vi "long_test_2.vi"(9 "string":string="tmp\\all_2.lvm", 10 "Instrument VISA in":T1={"AWG VISA"="81160A", "Oscilloscope  VISA "="DSO80204B", "Integration Board IP"="172.16.7.43", "connection ID"=refnum, "report out"=refnum, "report file path"=path "D:/CTA/Data_test"}, 11 "error in (no error)":errorcluster) -> (3 "error out":errorcluster)   [LabVIEW 2009]
uses:
  <vilib>/Utility/NIReport.llb/NI_report.lvclass
  <vilib>/Analysis/NI_AALBase.lvlib
panel:
  out "Numeric":i32
  out "atenuation":dbl[](array[numeric])
  out "clipping":dbl[](array[numeric])
  out "channel":dbl[](array[numeric])
  out "XY Graph":cluster{dbl[], dbl[]}[](graph)
  out "XY Graph 2":cluster{dbl[], dbl[]}[](graph)
  out "mean value 2":dbl=711.9915188935893
  in  "stop":bool
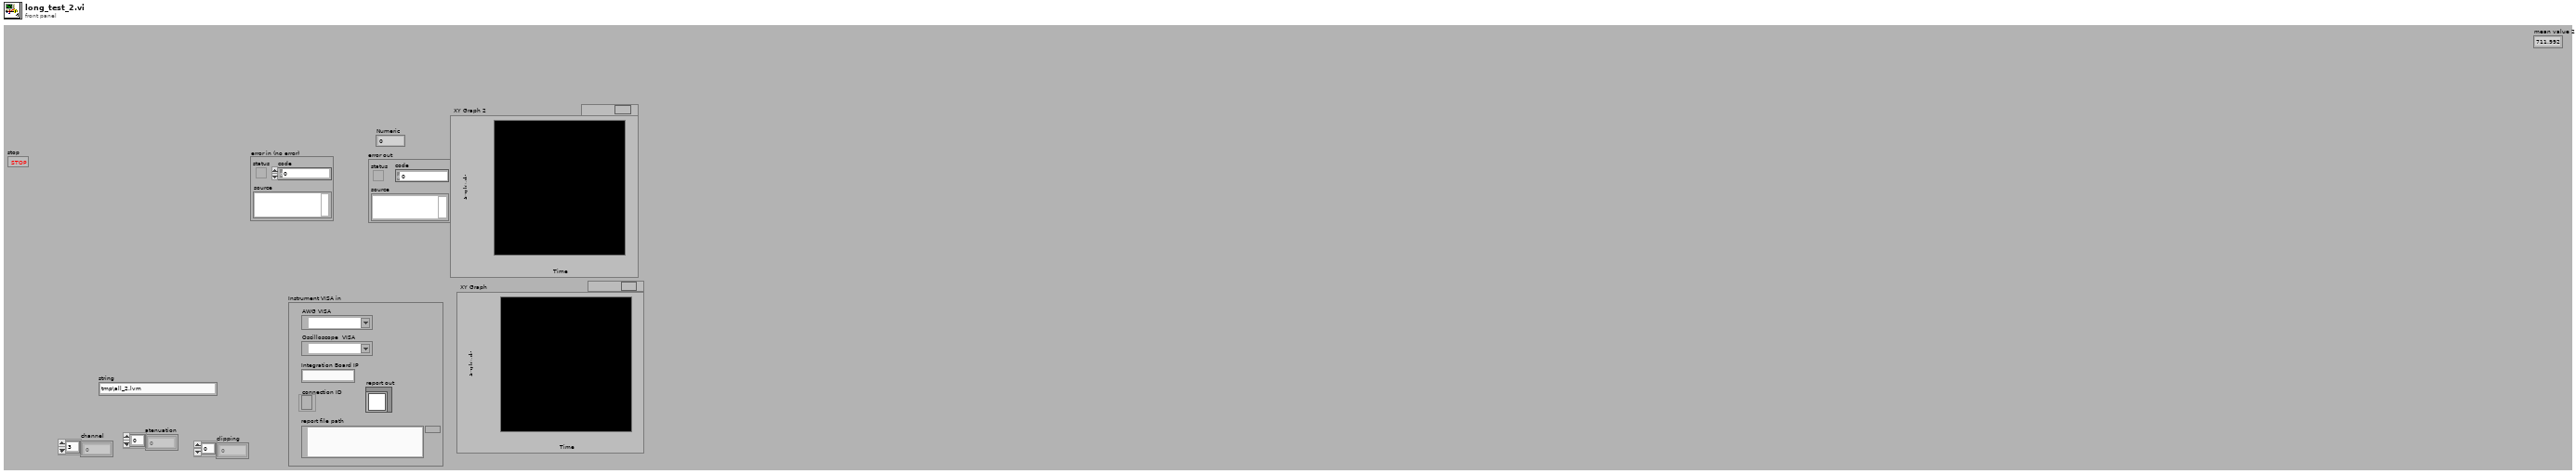
[diagram p1: front panel]
types:
  T1 = cluster{"AWG VISA":refnum<visa-resource-name>, "Oscilloscope  VISA ":refnum<visa-resource-name>, "Integration Board IP":string, "connection ID":refnum<k5>, "report out":refnum<class "NI_report.lvclass">, "report file path":path}
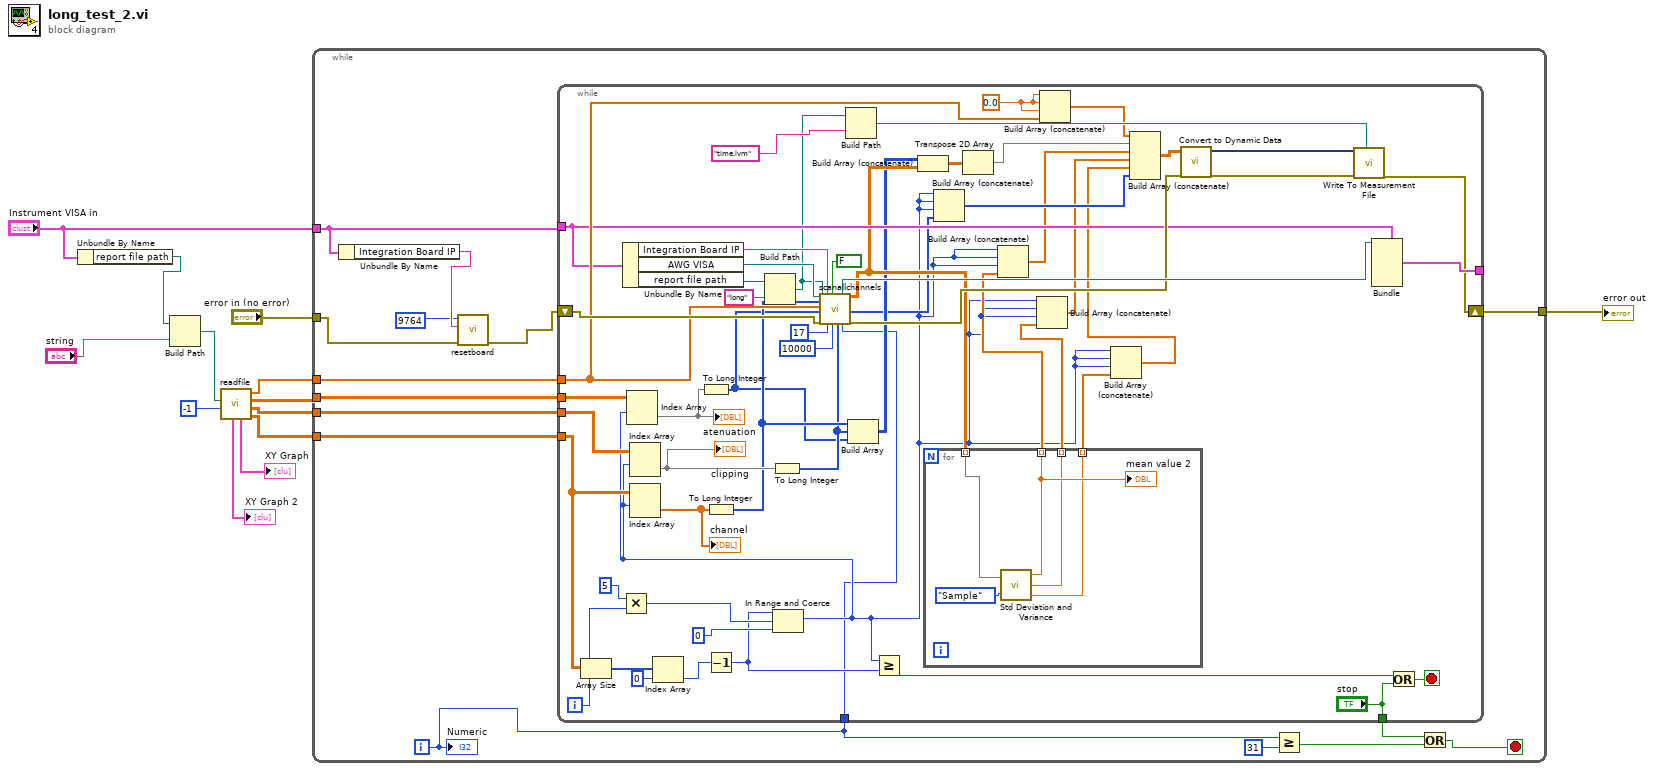
[diagram p0: block diagram]
diagram:
  n1 = Unbundle By Name("Instrument VISA in") -> ("report file path"=w5:path)
  n2 = Build Path(base path=w5, name or relative path="string") -> (appended path=w4:path)
  n3 = call "readfile.vi"("count"=-1, "file (use dialog)"=w4) -> ("channels"=w8:dbl[][], "clipping"=w7:dbl[][], "attenuator"=w6:dbl[][], "voltage"=w10:dbl[], "XY Graph"=→"XY Graph":cluster{dbl[], dbl[]}[], "XY Graph 2"=→"XY Graph 2":cluster{dbl[], dbl[]}[])  [unwired: 4 in]
  n4 = while {
    tunnel: w10 -> [w28]
    tunnel: "Instrument VISA in" -> [w21]
    tunnel: w8 -> [w27]
    tunnel: w7 -> [w26]
    tunnel: w6 -> [w25]
    tunnel: [w20] -> w2
    tunnel: "error in (no error)" -> [w19]
    i -> [w18]
    stop <- w14 stop-if-true
    n5 = Unbundle By Name(w21) -> ("Integration Board IP"=w24:string)
    n6 = call "resetboard.vi"("error in (no error)"=w19, "address"=w24, "remote port or service name"=u16 9764) -> ("error out"=w23:errorcluster)  [unwired: 7 in, 1 out]
    n7 = while {
      tunnel: w28 -> [w71]
      tunnel: w21 -> [w68]
      tunnel: [w69] -> _
      shift-right: [w65] -> w20
      shift-left: w23 -> [w75]
      tunnel: w27 -> [w62]
      tunnel: w26 -> [w63]
      tunnel: w25 -> [w64]
      tunnel: ["stop"] -> w16
      tunnel: w18 -> [w29]
      i -> [w36]
      stop <- w59 stop-if-true
      w76 = 0.0 ("element")
      n8 = Array Size(array=w62) -> (size(s)=w61:i32[])
      n9 = Multiply(x=5 ("index"), y=w36) -> (x*y=w32:i32)
      n10 = Unbundle By Name(w68) -> ("Integration Board IP"=w67:string, "AWG VISA"=w66:refnum<visa-resource-name>, "report file path"=w54:path)
      n11 = Index Array(array=w61, index=0) -> (element=w33:i32)
      n12 = Decrement(x=w33) -> (x-1=w30:i32)
      n13 = Build Path(base path=w54, name or relative path="long") -> (appended path=w53:path)
      n14 = In Range and Coerce(upper limit=w30, x=w32, lower limit=0) -> (coerced(x)=w31:i32)  [unwired: 1 out]
      n15 = Index Array(array=w64, index (row)=w31) -> (element=w55:dbl[])  [unwired: 1 in]
      "atenuation" <- w55
      n16 = Index Array(array=w63, index (row)=w31) -> (element=w57:dbl[])  [unwired: 1 in]
      "clipping" <- w57
      n17 = Index Array(array=w62, index (row)=w31) -> (element=w56:dbl[])  [unwired: 1 in]
      "channel" <- w56
      n18 = To Long Integer(number=w55) -> (32bit integer=w48:i32[])
      n19 = To Long Integer(number=w56) -> (32bit integer=w50:i32[])
      n20 = To Long Integer(number=w57) -> (32bit integer=w49:i32[])
      n21 = call "scanallchannels.vi"("VISA resource name in"=w66, "nm ch"=w50, "Voltages values"=w71, "Init ch value"=w48, "base path"=w53, "error in"=w75, "Integration Board IP"=w67, "L1 Address"=17, "Save test data"=FALSE, "Ch burst"=10000, "vclip"=w49, "Delay"=w29) -> ("VISA resource name out"=w81:refnum<visa-resource-name>, "L1  50%"=w47:dbl[][], "time"=w43:u32[], "error out"=w79:errorcluster)  [unwired: 3 in, 1 out]
      n22 = Build Path(base path=w53, name or relative path="time.lvm" ("string")) -> (appended path=w83:path)
      n23 = Build Array(w50, w49, w48) -> (w46:i32[][])
      n24 = Greater Or Equal?(x=w31, y=w30) -> (x >= y?=w58:bool)
      n25 = Build Array (concatenate)(w46, w47) -> (w45:dbl[][])
      n26 = for {
        tunnel: w47 -> [w88] mode=indexing
        tunnel: [w86] -> w41 mode=indexing
        tunnel: [w85] -> w40 mode=indexing
        tunnel: [w84] -> w38 mode=indexing
        n27 = call <vilib>:"Std Deviation and Variance.vi"("X"=w88, "Weighting (Sample)"=enum16{"Sample", "Population"}."Sample") -> ("mean"=w86:dbl, "standard deviation"=w85:dbl, "variance"=w84:dbl)
        "mean value 2" <- w86
      }
      n28 = Build Array (concatenate)(w31, w31, w31, w43) -> (w44:u32[])
      n29 = Transpose 2D Array(2D array=w45) -> (transposed array=w82:dbl[][])
      n30 = Build Array (concatenate)(w31, w31, w31, w41) -> (w42:dbl[])
      n31 = Build Array (concatenate)(w31, w31, w31, w40) -> (w39:dbl[])
      n32 = Build Array (concatenate)(w76, w76, w76, w71) -> (w77:dbl[])
      n33 = Build Array (concatenate)(w31, w31, w31, w38) -> (w37:dbl[])
      n34 = Build Array (concatenate)(w77, w82, w42, w39, w37, w44) -> (w80:dbl[][])
      n35 = call "Convert to Dynamic Data"("2D Array"=w80) -> ("Dynamic Data Type"=w78:dynamicdata)  [unwired: 3 in]
      n36 = call "Write To Measurement File"("Signals"=w78, "error in (no error)"=w79, "Filename"=w83) -> ("error out"=w65:errorcluster)  [unwired: 14 in, 2 out]
      n37 = Bundle(cluster=w68, "AWG VISA"=w81) -> (w69:T1)  [unwired: 5 in]
      n38 = Or(x=w58, y="stop") -> (x .or. y?=w59:bool)
    }
    n39 = Greater Or Equal?(x=w18, y=31) -> (x >= y?=w15:bool)
    n40 = Or(x=w16, y=w15) -> (x .or. y?=w14:bool)
    "Numeric" <- w18
  }
  "error out" <- w2
